vi "Log Write Loop.vi"(0 "Logging FIFO":refnum<k33>, 1 "Byte Stream File in":refnum<file>) -> ()   [LabVIEW 2014]
uses:
  Drive Train/Drive Metrics.ctl
  Drive Train/Drive States.ctl
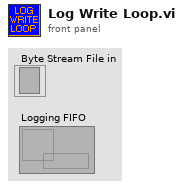
[diagram p1: front panel]
types:
  T1 = typedef "Drive Metrics.ctl" = cluster{"Timestamp":u32, "Drive State":T2, "Throttle":dbl, "Turn":dbl, "Heading":dbl, "Absolute Heading":dbl, "Left Velocity":dbl, "Left Encoder":dbl, "Right Velocity":dbl, "Right Encoder":dbl, "Left Power":dbl, "Right Power":dbl, "Last Shift":u32, "Shift Started":u32}
  T2 = typedef "Drive States.ctl" = enum16{"Initialize", "Low Gear", "Up Shift Begin", "Up Shifting", "Up Shift Delay", "High Gear", "Down Shift Begin", "Down Shifting", "Down Shift Delay"}
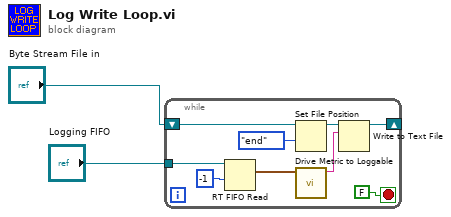
[diagram p0: block diagram]
diagram:
  n1 = while {
    tunnel: "Logging FIFO" -> [w11]
    shift-right: [w6] -> _
    shift-left: "Byte Stream File in" -> [w9]
    stop <- FALSE stop-if-true
    n2 = RT FIFO Read(0:w11, 2:-1 ("timeout in ms (0)")) -> (9:w5:T1)  [unwired: 2 in, 4 out]
    n3 = Set File Position(refnum=w9, from (0:start)=enum16{"start", "end", "current"}."end") -> (refnum out=w7:refnum<file>)  [unwired: 2 in, 1 out]
    n4 = call "Drive Metric to Loggable.vi"("Drive Metrics"=w5) -> ("resulting string"=w4:string)  [unwired: 10 in]
    n5 = Write to Text File(file (use dialog)=w7, text=w4) -> (refnum out=w6:refnum<file>)  [unwired: 2 in, 2 out]
  }
